vi "Get Queue Status.vi"(8 "error in (no error)":errorcluster, 11 "Priority Queue in":refnum<class "Priority Queue.lvclass">) -> (0 "error out":errorcluster, 1 "# pending insert":i32, 2 "# pending remove":i32, 3 "Priority Queue out":refnum<class "Priority Queue.lvclass">, 4 "# elements in queue":i32)   [LabVIEW 2020, in "Communicable State Machine.lvlib" / "Priority Queue.lvclass"]
uses:
  Priority Queue.lvclass
  Priority Queue.lvclass/Priority Queue.ctl
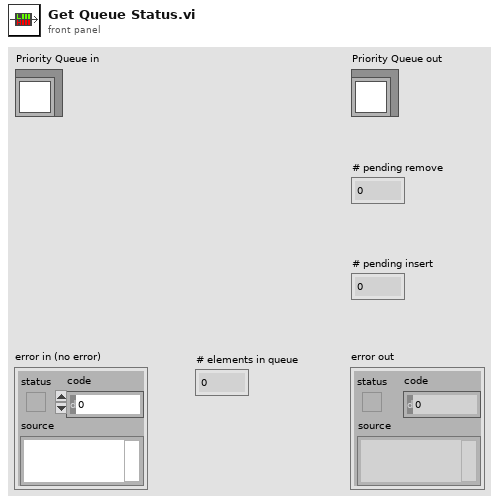
[diagram p1: front panel]
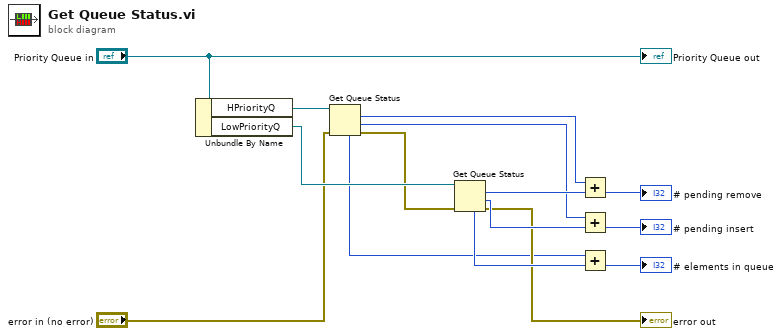
[diagram p0: block diagram]
diagram:
  n1 = Unbundle By Name("Priority Queue in") -> ("HPriorityQ"=w14:refnum<queue>, "LowPriorityQ"=w13:refnum<queue>)
  n2 = Get Queue Status(queue=w14, error in (no error)="error in (no error)") -> (# pending remove=w3:i32, # pending insert=w2:i32, error out=w9:errorcluster, # elements in queue=w1:i32)  [unwired: 1 in, 4 out]
  n3 = Get Queue Status(queue=w13, error in (no error)=w9) -> (# pending remove=w11:i32, # pending insert=w10:i32, error out=→"error out":errorcluster, # elements in queue=w12:i32)  [unwired: 1 in, 4 out]
  n4 = Add(x=w3, y=w11) -> (x+y=→"# pending remove":i32)
  n5 = Add(x=w2, y=w10) -> (x+y=→"# pending insert":i32)
  n6 = Add(x=w1, y=w12) -> (x+y=→"# elements in queue":i32)
  "Priority Queue out" <- "Priority Queue in"
